vi "calc results.vi"(0 "result in":T2, 7 "avg":waveform(dbl), 12 "time (s)":dbl, 13 "exec setpoint":dbl) -> (4 "result out":T2)   [LabVIEW 2019]
doc: "This is a Bug C(T) subVI.\n\nIt estimates the capacitance from the RC decay.\n\nPaul K Dixon\nP3600\nCSUSB Physics"
uses:
  typedefs/result.ctl
  typedefs/cap fit params.ctl
panel:
  in  "RC Fit":T1={"Resistance (Ohms)"=100000.0, "Est Time constant (s)"=0.0, "Est Capacitance (F)"=0.0} caption="RC Decay Fit"
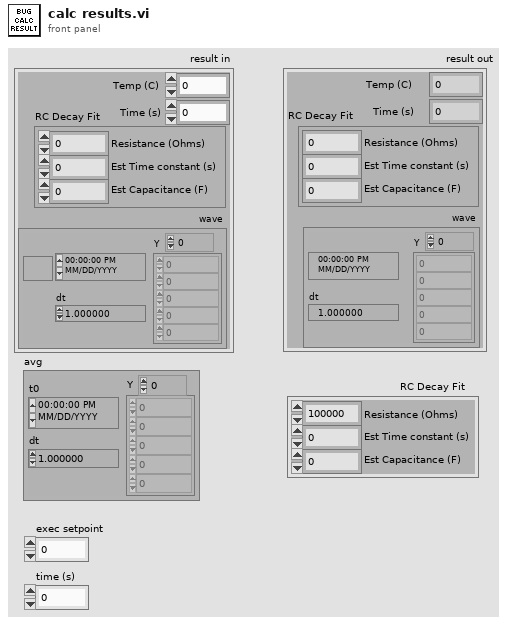
[diagram p1: front panel]
types:
  T1 = typedef "cap fit params.ctl" = cluster{"Resistance (Ohms)":dbl, "Est Time constant (s)":dbl, "Est Capacitance (F)":dbl}
  T2 = typedef "result.ctl" = cluster{"Temp (C)":dbl, "RC Fit":T1, "wave":waveform(dbl), "Time (s)":dbl}
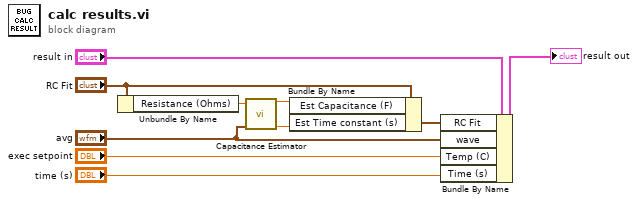
[diagram p0: block diagram]
diagram:
  n1 = Unbundle By Name("RC Fit") -> ("Resistance (Ohms)"=w7:dbl)
  n2 = call "Capacitance Estimator.vi"("Resistance (Ohms)"=w7, "normalized waveform"="avg") -> ("Estimated Capacitance (F)"=w4:dbl, "time constant (s)"=w3:dbl)  [unwired: 12 in]
  n3 = Bundle By Name(cluster="RC Fit", "Est Capacitance (F)"=w4, "Est Time constant (s)"=w3) -> (w5:T1)
  n4 = Bundle By Name(cluster="result in", "RC Fit"=w5, "wave"="avg", "Temp (C)"="exec setpoint", "Time (s)"="time (s)") -> (→"result out":T2)
